vi "clear Session Data.vi"(0 "Session in":refnum<class "Local Listener Session.lvclass">, 11 "error in":errorcluster) -> (4 "Session out":refnum<class "Local Listener Session.lvclass">, 15 "error out":errorcluster)   [LabVIEW 2012, in "REx.lvlib" / "Local Listener Session.lvclass"]
uses:
  Local Listener Session.lvclass
  <userlib>/_Session Fwk/Session - Root.lvclass
  Local Listener Session.lvclass/Local Listener Session.ctl
  Typedefs/Session Handle.ctl
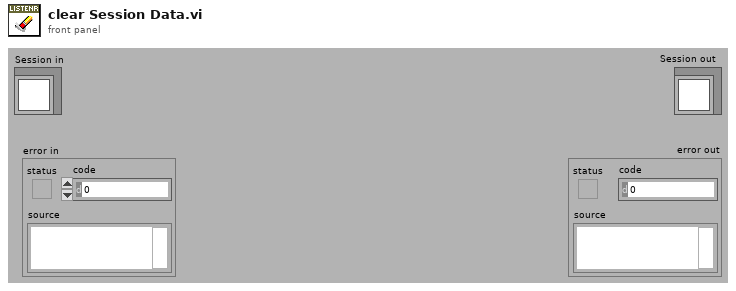
[diagram p1: front panel]
types:
  T1 = typedef "REx.lvlib/Local Listener Session.lvclass/Session Handle.ctl" = refnum<data-value>
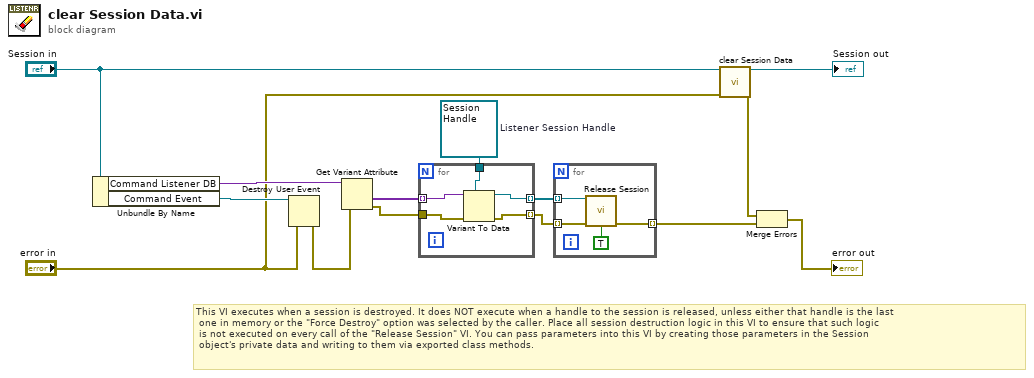
[diagram p0: block diagram]
diagram:
  w10 = T1 refnum  # Listener Session Handle
  # "This VI executes when a session is destroyed. It does NOT execute when a handle to the session is released, unless either that handle is the last\n one in memory or the \"Force Destroy\" option was selected by the caller. Place all session destruction logic in this VI to ensure that such logic\n is not executed on every call of the \"Release Session\" VI. You can pass parameters into this VI by creating those parameters in the Session \n object's private data and writing to them via exported class methods."
  n1 = Unbundle By Name("Session in") -> ("Command Listener DB"=w12:variant, "Command Event"=w5:refnum<user-event>)
  n2 = Destroy User Event(user event=w5, error in="error in") -> (error out=w4:errorcluster)
  n3 = Get Variant Attribute(Variant=w12, error in=w4) -> (values=w11:variant[], error out=w9:errorcluster)  [unwired: 2 in, 2 out]
  n4 = for {
    tunnel: w11 -> [w19] mode=indexing
    tunnel: w10 -> [w18]
    tunnel: [w15] -> w8 mode=indexing
    tunnel: w9 -> [w17]
    tunnel: [w16] -> w7 mode=indexing
    n5 = Variant To Data(error in=w17, type=w18, Variant=w19) -> (data=w15:T1, error out=w16:errorcluster)
  }
  n6 = for {
    tunnel: w8 -> [w23] mode=indexing
    tunnel: w7 -> [w22] mode=indexing
    tunnel: [w21] -> w6 mode=indexing
    n7 = call "Release Session.vi"("Session Handle"=w23, "error in (no error)"=w22, "force destroy? (F)"=TRUE) -> ("error out"=w21:errorcluster)  [unwired: 12 in]
  }
  n8 = call-parent "clear Session Data.vi"("OBJ - Measurement Session in"="Session in", "error in"="error in") -> ("OBJ - Measurement Session out"=→"Session out":refnum<class "Local Listener Session.lvclass">, "error out"=w2:errorcluster)  [unwired: 12 in]
  n9 = Merge Errors(w2, w6) -> (→"error out":errorcluster)
